vi "LoadGraphics.vi"(4 "Templates user event":refnum<user-event>, 6 "Glyphs user event":refnum<user-event>, 8 "error in":errorcluster, 9 "Source":T1=enum."Icon Templates VI", 10 "Check Template?":bool, 11 "Graphic Root Folder":path) -> (0 "error out":errorcluster, 3 "Glyphs":T2[](array[typedef]), 5 "Match?":bool, 7 "Match Index":i32)   [LabVIEW 2020]
uses:
  vi.lib/LabVIEW Icon API/lv_icon/Controls/Graphic.ctl
  vi.lib/LabVIEW Icon API/lv_icon/lv_icon.lvlib
  Controls/IconFilename.ctl
  Controls/Path&Icon.ctl
  vi.lib/LabVIEW Icon API/lv_icon/Controls/Pathes.ctl
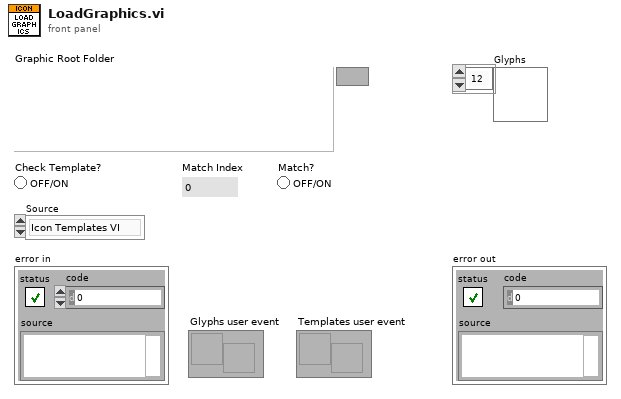
[diagram p1: front panel]
types:
  T1 = typedef "Pathes.ctl" = enum16{"Root Path", "Icon Templates", "Icon Templates VI", "Icon Templates Lib", "Glyphs"}
  T2 = typedef "Path&Icon.ctl" = cluster{"Rectangle":cluster{"left":i16, "top":i16, "right":i16, "bottom":i16}, "Path":path, "Image":picture, "Filter":string, "FileName":string}
  T3 = typedef "IconFilename.ctl" = cluster{"Name":string, "File Extension  ":string, "Filter":string, "Path":path}
  T4 = typedef "Graphic.ctl" = cluster{"Rectangle":cluster{"left":i16, "top":i16, "right":i16, "bottom":i16}, "Path":path, "Image":picture, "Filter":string, "FileName":string}
  T5 = typedef "LabVIEW Icon Stored Information.ctl" = cluster{"Text Visible?":bool, "Text Opacity":u8, "Templ Visible?":bool, "Templ Opacity":u8, "Relative Path from 1 to 2":path, "Image":picture, "All User Layers":refnum<class "Layer.lvclass">[], "Body Text":T6}
  T6 = typedef "BodyText.ctl" = cluster{"Line 1 text":string, "Line 2 text":string, "Line 3 text":string, "Line 4 text":string, "Line 1 color":u32, "Line 2 color":u32, "Line 3 color":u32, "Line 4 color":u32, "Body Text Spec":cluster{"Font":T7, "Alignment":T8, "Size":u8}, "Center text vertically":bool, "Capitalize Text":bool}
  T7 = typedef "Font.ctl" = string
  T8 = typedef "Alignment.ctl" = u16
  T9 = typedef "imagedata.ctl" = cluster{"image type":i32, "image depth":i32, "image":u8[], "mask":u8[], "colors":u32[], "Rectangle":cluster{"left":i16, "top":i16, "right":i16, "bottom":i16}}
  T10 = cluster{"left":i16, "top":i16, "right":i16, "bottom":i16}
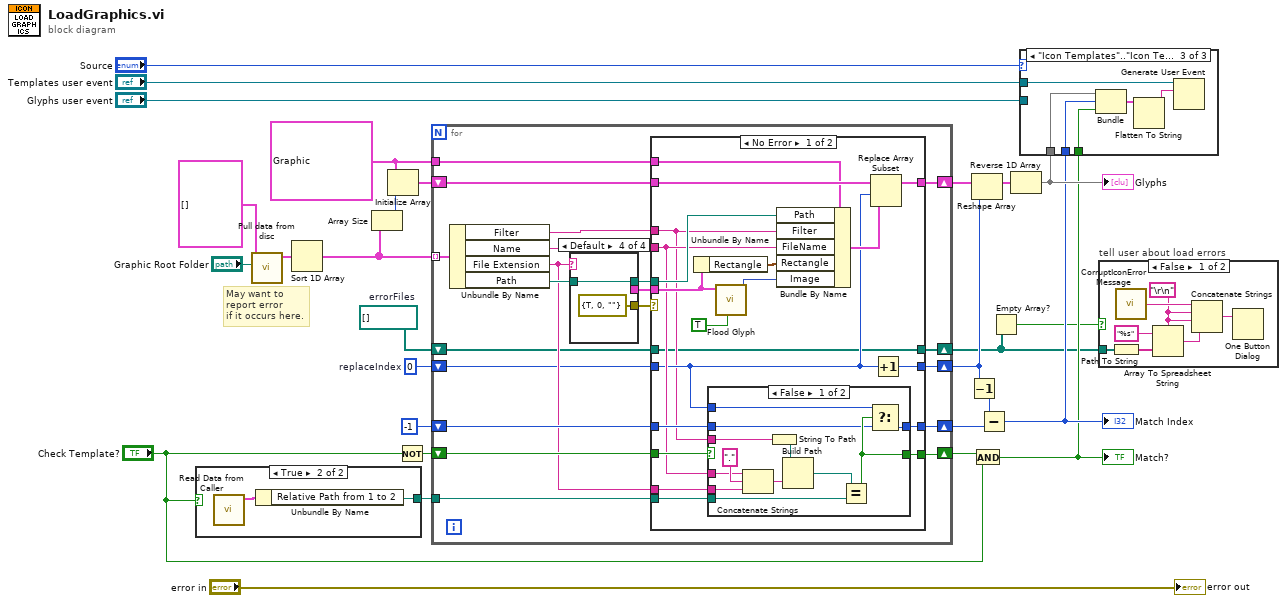
[diagram p0: block diagram]
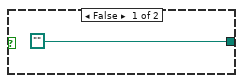
[diagram p3: hidden frame]
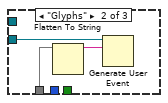
[diagram p5: hidden frame]
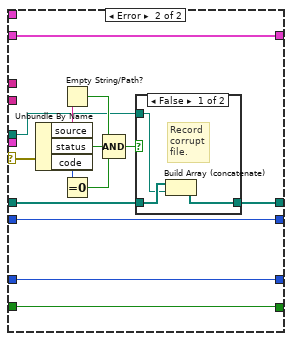
[diagram p7: hidden frame]
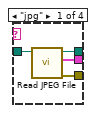
[diagram p9: hidden frame]
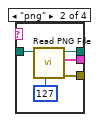
[diagram p10: hidden frame]
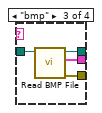
[diagram p11: hidden frame]
diagram:
  w6 = 0  # replaceIndex
  w7 = path[] []  # errorFiles
  w9 = T4 {"Rectangle"={"left"=0, "top"=0, "right"=0, "bottom"=0}, "Path"=path "", "Image"=bytes[0], "Filter"="", "FileName"=""} ("Path & Icon")
  # "May want to\nreport error\nif it occurs here."
  n1 = case shown="True" "Check Template?" {
    tunnel: [path "" w30] -> w12
    frame False {
    }
    frame True {
      n2 = call "Read Data from Caller.vi"() -> ("data"=w31:T5)  [unwired: 3 in, 8 out]
      n3 = Unbundle By Name(w31) -> ("Relative Path from 1 to 2"=w30:path)
    }
  }
  n4 = call "Pull data from disc.vi"("Graphic Root Folder"="Graphic Root Folder", "Data in"=T3[] []) -> ("Data out"=w11:T3[])  [unwired: 1 in, 8 out]
  n5 = Sort 1D Array(array=w11) -> (sorted array=w27:T3[])
  n6 = Array Size(array=w27) -> (size(s)=w28:i32)
  n7 = Initialize Array(w9, w28) -> (w26:T4[])
  n8 = Not(x="Check Template?") -> (.not. x?=w24:bool)
  n9 = for {
    tunnel: w27 -> [w51] mode=indexing
    shift-right: [w32] -> w1
    shift-left: w7 -> [w33]
    shift-right: [w48] -> w25
    shift-left: w26 -> [w49]
    shift-right: [w44] -> w19
    shift-left: w24 -> [w47]
    tunnel: w12 -> [w45]
    shift-right: [w43] -> w22
    shift-left: -1 -> [w42]
    tunnel: w9 -> [w38]
    shift-right: [w36] -> w3
    shift-left: w6 -> [w37]
    n10 = Unbundle By Name(w51) -> ("Filter"=w35:string, "Name"=w40:string, "File Extension"=w39:string, "Path"=w50:path)
    n11 = case shown="Default" w39 {
      tunnel: [w107 w112 w116 errorcluster {"status"=TRUE, "code"=0, "source"=""} ("error out")] -> w34
      tunnel: [w106 w111 w115 _] -> w41
      tunnel: [w104 w109 w113 w118] -> w46
      tunnel: w50 -> [w105 w110 w114 w118]
      frame "jpg" {
        n12 = call <vilib>:"Read JPEG File.vi"("path to JPEG file"=w105) -> ("error out"=w107:errorcluster, "image data"=w106:T9, "path"=w104:path)  [unwired: 1 in, 7 out]
      }
      frame "png" {
        n13 = call <vilib>:"Read PNG File.vi"("Transparency Thresh"=u8 127, "path to PNG file"=w110) -> ("error out"=w112:errorcluster, "image data"=w111:T9, "path"=w109:path)  [unwired: 1 in, 6 out]
      }
      frame "bmp" {
        n14 = call <vilib>:"Read BMP File.vi"("path to BMP file"=w114) -> ("error out"=w116:errorcluster, "image data"=w115:T9, "path"=w113:path)  [unwired: 1 in, 7 out]
      }
      frame Default {
      }
    }
    n15 = case shown="No Error" w34 {
      selector: w34 -> [_ w98]
      tunnel: w49 -> [w71 w99]
      tunnel: [w70 w99] -> w48
      tunnel: w47 -> [w68 w93]
      tunnel: w46 -> [w67 w86]
      tunnel: w45 -> [w66 _]
      tunnel: [w65 w93] -> w44
      tunnel: [w64 w94] -> w43
      tunnel: w42 -> [w63 w94]
      tunnel: w41 -> [w62 _]
      tunnel: w40 -> [w61 _]
      tunnel: w39 -> [w60 _]
      tunnel: w38 -> [w59 _]
      tunnel: w37 -> [w58 w95]
      tunnel: [w57 w95] -> w36
      tunnel: w35 -> [w55 _]
      tunnel: w33 -> [w53 w91]
      tunnel: [w53 w87] -> w32
      frame No Error {
        n16 = Unbundle By Name(w62) -> ("Rectangle"=w54:T10)
        n17 = case shown="False" w68 {
          selector: w68 -> [_ w85]
          tunnel: w66 -> [w83 _]
          tunnel: [w81 w85] -> w65
          tunnel: [w82 w84] -> w64
          tunnel: w58 -> [w80 _]
          tunnel: w63 -> [w79 w84]
          tunnel: w55 -> [w74 _]
          tunnel: w61 -> [w73 _]
          tunnel: w60 -> [w72 _]
          frame False {
            n18 = Concatenate Strings(w73, "." ("string"), w72) -> (w78:string)
            n19 = String To Path(string=w74) -> (path=w76:path)
            n20 = Build Path(base path=w76, name or relative path=w78) -> (appended path=w75:path)
            n21 = Equal?(x=w75, y=w83) -> (x = y?=w81:bool)
            n22 = Select(t=w80, s=w81, f=w79) -> (s? t:f=w82:i32)
          }
          frame True {
          }
        }
        n23 = call "Flood Glyph.vi"("Use New Fill Algorithm? (F)"=TRUE, "image data"=w62) -> ("Pic Out"=w56:picture)  [unwired: 9 out]
        n24 = Bundle By Name(cluster=w59, "Path"=w67, "Filter"=w55, "FileName"=w61, "Rectangle"=w54, "Image"=w56) -> (w69:T4)
        n25 = Replace Array Subset(array=w71, new element=w69, index=w58) -> (w70:T4[])
        n26 = Increment(x=w58) -> (x+1=w57:i32)
      }
      frame Error {
        n27 = Unbundle By Name(w98) -> ("source"=w97:string, "status"=w89:bool, "code"=w96:i32)
        n28 = Empty String/Path?(string/path=w97) -> (empty?=w92:bool)
        n29 = Equal To 0?(x=w96) -> (x = 0?=w90:bool)
        n30 = Compound Arithmetic op=AND(w92, w89, w90) -> (w88:bool)
        n31 = case shown="False" w88 {
          tunnel: w91 -> [w102 w103]
          tunnel: [w100 w103] -> w87
          tunnel: w86 -> [w101 _]
          frame False {
            # "Record\ncorrupt\nfile."
            n32 = Build Array (concatenate)(w102, w101) -> (w100:path[])
          }
          frame True {
            # "Unsupported\nfile\nextension -\nignore it."
          }
        }
      }
    }
  }
  n33 = Decrement(x=w3) -> (x-1=w5:i32)
  n34 = Reshape Array(w25, w3) -> (w4:T4[])
  n35 = And(x=w19, y="Check Template?") -> (x .and. y?=w18:bool)
  "Match?" <- w18
  n36 = Subtract(x=w5, y=w22) -> (x-y=w20:i32)
  "Match Index" <- w20
  n37 = Empty Array?(array=w1) -> (empty?=w2:bool)
  n38 = Reverse 1D Array(array=w4) -> (reversed array=w21:T4[])
  "Glyphs" <- w21
  n39 = case shown="\"Icon Templates\"..\"Icon Templates Lib\"" "Source" {
    tunnel: w21 -> [_ w120 w124]
    tunnel: w20 -> [_ _ w123]
    tunnel: w18 -> [_ _ w126]
    tunnel: "Glyphs user event" -> [_ w119 _]
    tunnel: "Templates user event" -> [_ _ w122]
    frame "Root Path", Default {
    }
    frame "Glyphs" {
      n40 = Flatten To String(anything=w120) -> (data string=w121:string)  [unwired: 1 in, 4 out]
      n41 = Generate User Event(user event=w119, event data cluster=w121) -> ()  [unwired: 2 in, 2 out]
    }
    frame "Icon Templates".."Icon Templates Lib" {
      n42 = Bundle(w124, w123, w126) -> (w125:cluster{T4[], i32, bool})  [unwired: 1 out]
      n43 = Flatten To String(anything=w125) -> (data string=w127:string)  [unwired: 1 in, 4 out]
      n44 = Generate User Event(user event=w122, event data cluster=w127) -> ()  [unwired: 2 in, 2 out]
    }
  }
  n45 = case "tell user about load errors" shown="False" w2 {
    tunnel: w1 -> [w133 _]
    frame False {
      w131 = "\r\n"
      n46 = Path To String(path=w133) -> (string=w128:string[])
      n47 = call "CorruptIconErrorMessage.vi"() -> ("corruptIconErrorMsg"=w134:string)  [unwired: 1 in]
      n48 = Array To Spreadsheet String(delimiter (Tab)=w131, array=w128, 3:"%s" ("format string")) -> (spreadsheet string=w130:string)
      n49 = Concatenate Strings(w134, w131, w131, w130) -> (w129:string)
      n50 = One Button Dialog(message=w129) -> ()  [unwired: 1 in, 1 out]
    }
    frame True {
    }
  }
  "error out" <- "error in"
